vi "readFromXML.vi"(8 "error in (no error)":errorcluster, 10 "XML in":string, 11 "AzElTarget in":refnum<class "AzElTarget.lvclass">) -> (0 "error out":errorcluster, 3 "AzElTarget out":refnum<class "AzElTarget.lvclass">)   [LabVIEW 2022 SP3, in "TCSDataDefinitions.lvlib" / "TCSCommand.lvlib" / "TargetConfiguration.lvlib" / "Target.lvlib" / "FixedTarget.lvlib" / "AzElTarget.lvclass"]
uses:
  AzElTarget.lvclass
  AzElTarget.lvclass/AzElTarget.ctl
  FixedTarget/FixedTarget.lvclass
  AzElParameters/AzElParameters.lvclass
  <userlib>/Common/XML/XMLParser/XMLParser.lvclass
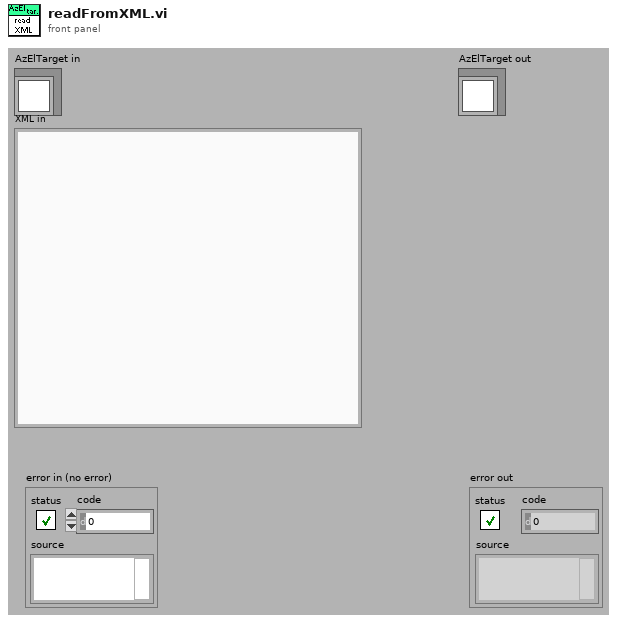
[diagram p1: front panel]
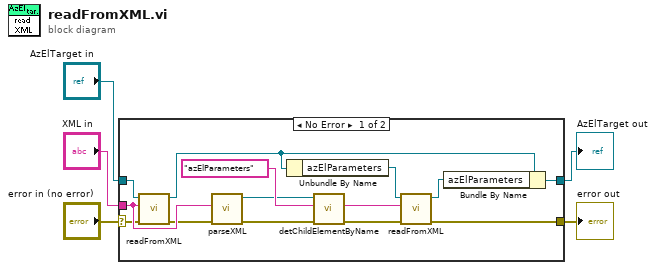
[diagram p0: block diagram]
diagram:
  n1 = case shown="No Error" "error in (no error)" {
    selector: "error in (no error)" -> [w10 w21]
    tunnel: [w15 w21] -> w4
    tunnel: [w11 w20] -> w2
    tunnel: "AzElTarget in" -> [w13 w20]
    tunnel: "XML in" -> [w12 _]
    frame No Error {
      n2 = call-parent "readFromXML.vi"("error in (no error)"=w10, "XMLin"=w12, "FixedTarget in"=w13) -> ("error out"=w9:errorcluster, "FixedTarget out"=w7:refnum<class "AzElTarget.lvclass">)  [unwired: 7 in]
      n3 = call <userlib>:"parseXML.vi"("error in (no error)"=w9, "XMLString in"=w12) -> ("error out"=w18:errorcluster, "Element out"=w6:refnum<class "XMLParser.lvclass">)  [unwired: 8 in]
      n4 = Unbundle By Name(w7) -> ("azElParameters"=w8:refnum<class "AzElParameters.lvclass">)
      n5 = call <userlib>:"detChildElementByName.vi"("error in (no error)"=w18, "childName"="azElParameters" ("ChildName"), "Element in"=w6) -> ("error out"=w16:errorcluster, "childXML"=w17:string)  [unwired: 5 in, 2 out]
      n6 = call-dynamic "readFromXML.vi"("error in (no error)"=w16, "XMLin"=w17, "AzElParameters in"=w8) -> ("error out"=w15:errorcluster, "AzElParameters out"=w14:refnum<class "AzElParameters.lvclass">)  [unwired: 7 in]
      n7 = Bundle By Name(cluster=w7, "azElParameters"=w14) -> (w11:refnum<class "AzElTarget.lvclass">)
    }
    frame Error {
    }
  }
  "error out" <- w4
  "AzElTarget out" <- w2
